vi "ReachedCountsInTime.vi"() -> ()   [LabVIEW 2016]
panel:
  in  "Input":bool
  in  "Count":i32
  in  "Time Limit":u32
  out "Output":bool
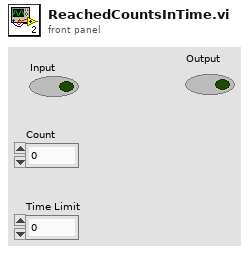
[diagram p1: front panel]
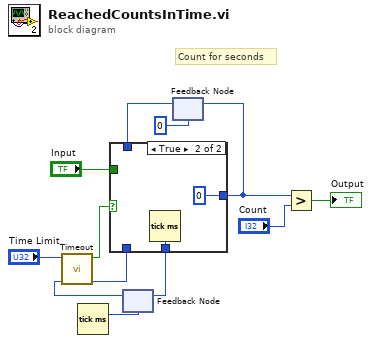
[diagram p0: block diagram]
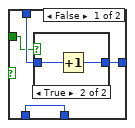
[diagram p2: hidden frame]
diagram:
  # "Count for seconds"
  n1 = Tick Count (ms)() -> (millisecond timer value=w12:u32)
  n2 = feedback #1(w12) -> (w10:u32)
  n3 = call "Timeout.vi"("Start Time In"=w10, "Time Limit"="Time Limit") -> ("Start Time Out"=w3:u32, "Timeout"=w9:bool)  [unwired: 8 in]
  n4 = feedback #2(0) -> (w7:i32)
  n5 = case shown="True" w9 {
    tunnel: [w15 0] -> w6
    tunnel: w7 -> [w16 _]
    tunnel: "Input" -> [w14 _]
    tunnel: w3 -> [w13 _]
    tunnel: [w13 w20] -> w2
    frame False {
      n6 = case shown="True" w14 {
        tunnel: w16 -> [w17 w18]
        tunnel: [w17 w19] -> w15
        frame False {
        }
        frame True {
          n7 = Increment(x=w18) -> (x+1=w19:i32)
        }
      }
    }
    frame True {
      n8 = Tick Count (ms)() -> (millisecond timer value=w20:u32)
    }
  }
  n9 = feedback-in #1(w2) -> ()
  n10 = feedback-in #2(w6) -> ()
  n11 = Greater?(x=w6, y="Count") -> (0:→"Output":bool)
